vi "StartTask.vi"(8 "error in (no error)":errorcluster, 11 "NI_DAQmx(AI) in":refnum<class "NI_DAQmx(AI).lvclass">) -> (0 "error out":errorcluster, 3 "NI_DAQmx(AI) out":refnum<class "NI_DAQmx(AI).lvclass">)   [LabVIEW 2025, in "NI_DAQmx(AI).lvclass"]
uses:
  NI_DAQmx(AI).lvclass
  NI_DAQmx(AI).lvclass/NI_DAQmx(AI).ctl
  DAQ_Abstr/Task_Type/AI_Task/AI_Task/AI_Task.lvclass
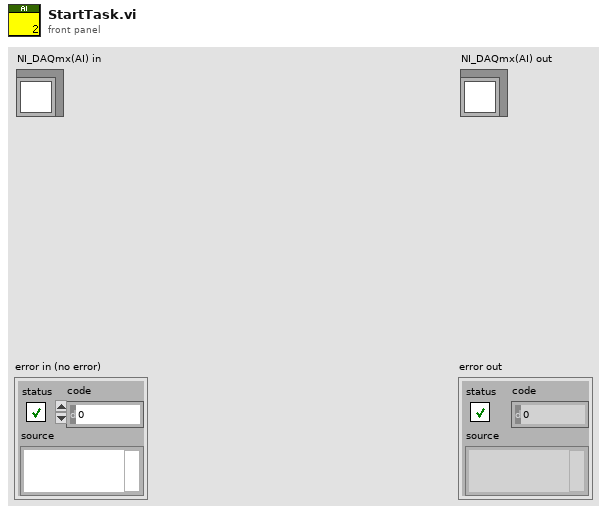
[diagram p1: front panel]
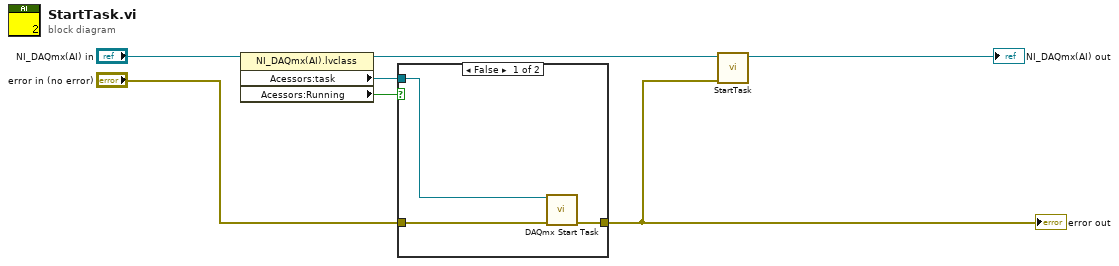
[diagram p0: block diagram]
diagram:
  n1 = property class="NI_DAQmx(AI).lvclass"(reference="NI_DAQmx(AI) in") -> (reference out=w4:refnum<class "NI_DAQmx(AI).lvclass">, "Acessors:task"=w7:refnum<k21>, "Acessors:Running"=w1:bool)  [unwired: 1 in, 1 out]
  n2 = case shown="False" w1 {
    tunnel: w7 -> [w10 _]
    tunnel: "error in (no error)" -> [w9 w11]
    tunnel: [w8 w11] -> w2
    frame False {
      n3 = call <vilib>:"DAQmx Start Task.vi"("task/channels in"=w10, "error in"=w9) -> ("error out"=w8:errorcluster)  [unwired: 12 in, 1 out]
    }
    frame True {
    }
  }
  "error out" <- w2
  n4 = call-parent "StartTask.vi"("error in (no error)"=w2, "Task_Abstr in"=w4) -> ("Task_Abstr out"=→"NI_DAQmx(AI) out":refnum<class "NI_DAQmx(AI).lvclass">)  [unwired: 8 in, 1 out]
